vi "Test MFC Step Response.vi"() -> ()   [LabVIEW 2013]
doc: "This VI gets the step response of the 500 SLPM mass flow controller controlling the air flow through the system. It records the pressure readings directly from the static pressure sensor just down stream of the sintered plate in the combustor.\n\nIt can also be used to test the fuel mass flow controllers by selecting the fuel line using the enum on the front panel and then inputting a voltage to the MFC. No pressure sensors are attached to the fuel MFCs."
uses:
  Controls/mfc_enable_boolean_cluster.ctl
  Controls/mfc_voltage_cluster.ctl
  <vilib>/DAQmx/write.llb/DAQmx Write (Digital 1D Bool NChan 1Samp 1Line).vi
  <vilib>/DAQmx/write.llb/DAQmx Write (Analog 1D DBL NChan 1Samp).vi
  <vilib>/DAQmx/read.llb/DAQmx Read (Analog 1D DBL NChan 1Samp).vi
  <vilib>/DAQmx/read.llb/DAQmx Read (Analog 2D DBL NChan NSamp).vi
  <vilib>/DAQmx/miscellaneous.llb/DAQmx Fill In Error Info.vi
  <vilib>/Analysis/NI_AALPro.lvlib
  <resource>/objmgr/daqmx.rc
  <vilib>/ptbypt/NI_PtbyPt.lvlib
panel:
  out "Flame?":bool
  out "Elapsed Time (s)":dbl
  in  "End":bool
  out "Remaining":dbl caption="Time to Shutdown"
  out "Over Temp?":T1 caption="Over Temperature"
  in  "Save Data?":bool
  in  "MFC Voltage":T2 {"Outer" scale=0.0..5.0; "Middle" scale=0.0..5.0; "Pilot" scale=0.0..5.0; "Air" scale=0.0..5.0}
  in  "MFC Enable":T3
  out "Pressure Response":T4(graph)
  in  "Stop Button":bool
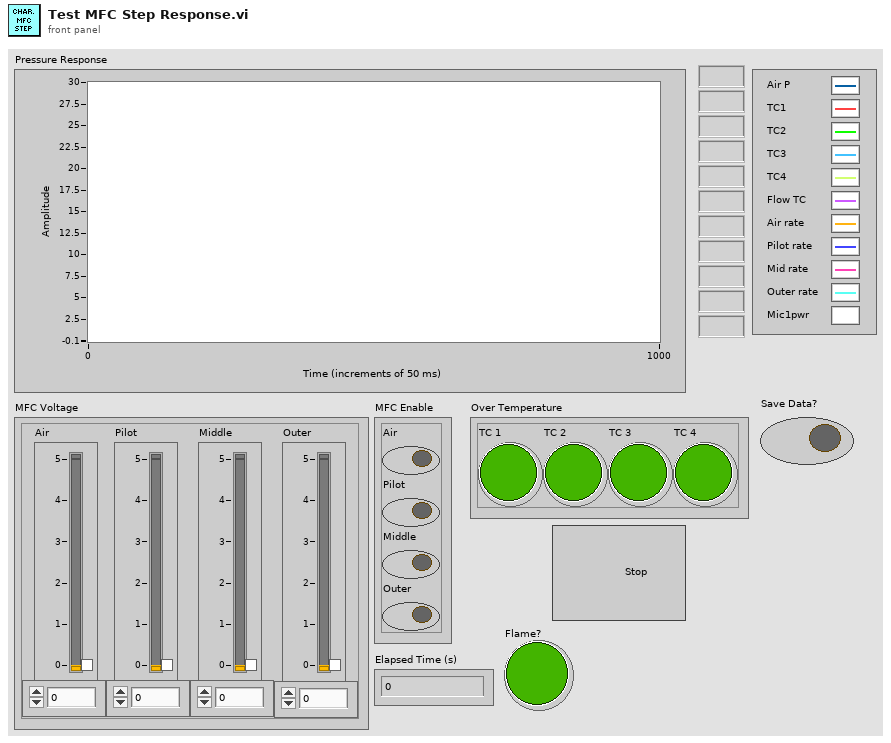
[diagram p1: front panel]
types:
  T1 = cluster{"TC 1":bool, "TC 2":bool, "TC 3":bool, "TC 4":bool}
  T2 = typedef "mfc_voltage_cluster.ctl" = cluster{"Air":dbl, "Pilot":dbl, "Middle":dbl, "Outer":dbl}
  T3 = typedef "mfc_enable_boolean_cluster.ctl" = cluster{"Air":bool, "Pilot":bool, "Middle":bool, "Outer":bool}
  T4 = cluster{"[0]":dbl, "[1]":dbl, "[2]":dbl, "[3]":dbl, "[4]":dbl, "[5]":dbl, "[6]":dbl, "[7]":dbl, "[8]":dbl, "[9]":dbl, "[10]":dbl}
  T5 = enum16{"open", "replace", "create", "open or create", "replace or create", "replace or create with confirmation"}
  T6 = cluster{"[0]":bool, "[1]":bool, "[2]":bool, "[3]":bool}
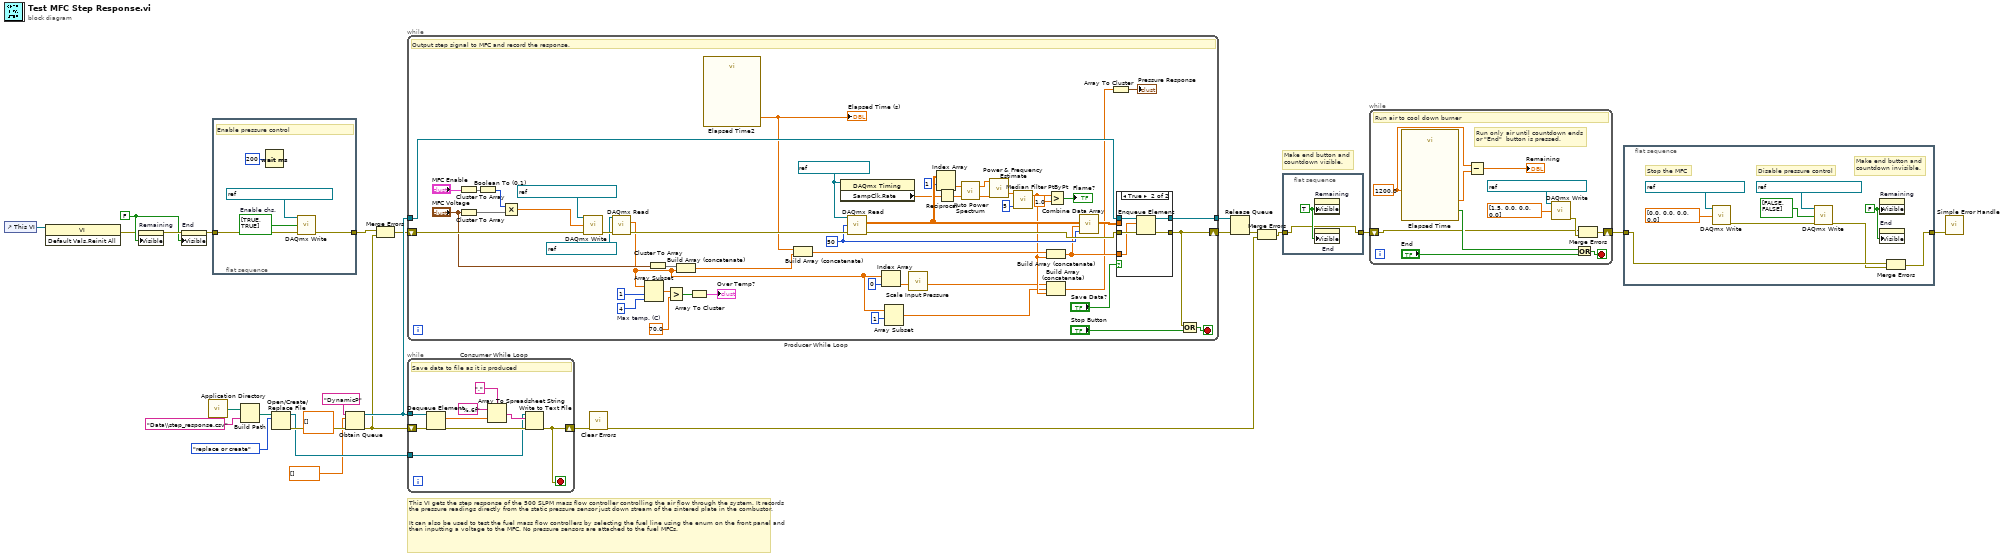
[diagram p0: block diagram]
diagram:
  (unwired) dbl[][] [] ("data")
  w23 = FALSE ("Visible")
  # "Make end button and\ncountdown visible."
  # "This VI gets the step response of the 500 SLPM mass flow controller controlling the air flow through the system. It records the pressure readings directly from the static pressure sensor just down stream of the sintered plate in the combustor.\n\nIt can also be used to test the fuel mass flow controllers by selecting the fuel line using the enum on the front panel and then inputting a voltage to the MFC. No pressure sensors are attached to the fuel MFCs."
  n1 = control-ref of="This VI"() -> (w26:refnum<vi>)
  n2 = invoke class="VI" method="Default Vals.Reinit All"(reference=w26) -> (error out=w18:errorcluster)  [unwired: 2 in, 2 out]
  n3 = property on="Remaining" class="DigNum (strict)"(error in=w18, "Visible"=w23) -> (error out=w25:errorcluster)  [unwired: 1 in, 1 out]
  n4 = property on="End" class="Bool"(error in=w25, "Visible"=w23) -> (error out=w24:errorcluster)  [unwired: 1 in, 1 out]
  n5 = call <vilib>:"Application Directory.vi"() -> ("Application Directory"=w14:path)
  n6 = flat-sequence {
    tunnel: [w29] -> w20
    tunnel: w24 -> [w27]
    frame #0 {
      w28 = bool[] [TRUE, TRUE]  # Enable chs.
      # "Enable pressure control"
      n7 = Wait (ms)(milliseconds to wait=u32 200) -> ()  [unwired: 1 out]
      n8 = call-poly <vilib>:"DAQmx Write.vi"("task/channels in"=refnum<k21> "MFCOutputEnable_S2P0L67", "data"=w28, "error in"=w27) -> ("error out"=w29:errorcluster)  [unwired: 10 in, 2 out]
    }
  }
  n9 = Build Path(base path=w14, name or relative path="Data\\step_response.csv") -> (appended path=w8:path)
  n10 = Open/Create/Replace File(file path (use dialog)=w8, operation (0:open)=T5."replace or create") -> (refnum out=w7:refnum<file>, error out=w9:errorcluster)  [unwired: 4 in, 1 out]
  n11 = Obtain Queue(name (unnamed)="DynamicP", element data type=dbl[] [], error in (no error)=w9) -> (queue out=w21:refnum<queue>, error out=w12:errorcluster)  [unwired: 2 in, 1 out]
  n12 = Merge Errors(w20, w12) -> (w19:errorcluster)
  n13 = while "Producer While Loop" {
    shift-right: [w66] -> w16
    shift-left: w19 -> [w75]
    tunnel: w21 -> [w67]
    tunnel: [w65] -> w15
    stop <- w80 stop-if-true
    w63 = 50 ("number of samples per channel")
    w50 = refnum<k21> "DynP_all_S6AI0-4" ("task/channels in")
    w72 = 70.0  # Max temp. (C)
    # "Output step signal to MFC and record the response."
    n14 = Cluster To Array(cluster="MFC Enable") -> (array=w78:bool[])
    n15 = Cluster To Array(cluster="MFC Voltage") -> (array=w77:dbl[])
    n16 = Boolean To (0,1)(Boolean=w78) -> (0, 1=w76:i16[])
    n17 = Multiply(x=w76, y=w77) -> (x*y=w38:dbl[])
    n18 = call-poly <vilib>:"DAQmx Write.vi"("task/channels in"=refnum<k21> "MFCVoltageOut_S2AO0-3", "data"=w38, "error in"=w75) -> ("error out"=w74:errorcluster)  [unwired: 10 in, 2 out]
    n19 = call-poly <vilib>:"DAQmx Read.vi"("task/channels in"=refnum<k21> "AiTasks_TC_P_S3" ("DAQmx Task Name"), "error in"=w74) -> ("data"=w35:dbl[], "error out"=w71:errorcluster)  [unwired: 11 in, 1 out]
    n20 = Array Subset(array=w35, index=1, length=4) -> (w58:dbl[])
    n21 = Cluster To Array(cluster="MFC Voltage") -> (array=w69:dbl[])
    n22 = Greater?(x=w58, y=w72) -> (0:w57:bool[])
    n23 = Build Array (concatenate)(w69, w35) -> (w60:dbl[])
    n24 = Array To Cluster(array=w57) -> (cluster=→"Over Temp?":T6)
    n25 = call "Elapsed Time2"() -> ("Elapsed Time (s)"=w61:dbl)  [unwired: 12 in, 7 out]
    "Elapsed Time (s)" <- w61
    n26 = Build Array (concatenate)(w61, w60) -> (w55:dbl[])
    n27 = property class="DAQmx Timing"(reference=w50) -> ("SampClk.Rate"=w49:dbl)  [unwired: 1 in, 2 out]
    n28 = call-poly <vilib>:"DAQmx Read.vi"("task/channels in"=w50, "number of samples per channel"=w63, "error in"=w71) -> ("data"=w53:dbl[][], "error out"=w83:errorcluster)  [unwired: 10 in, 1 out]
    n29 = Index Array(array=w35, index=0) -> (element=w36:dbl)
    n30 = Array Subset(array=w35, index=1) -> (w32:dbl[])  [unwired: 1 in]
    n31 = call "Scale Input Pressure.vi"("Pressure (V)"=w36) -> ("Pressure (psi atm)"=w33:dbl)  [unwired: 10 in]
    n32 = Index Array(array=w53, index (row)=1) -> (element=w51:dbl[])  [unwired: 1 in]
    n33 = Reciprocal(x=w49) -> (1/x=w48:dbl)
    n34 = call <vilib>:"Auto Power Spectrum.vi"("dt"=w48, "Signal (V)"=w51) -> ("df"=w46:dbl, "Power Spectrum (V^2 rms)"=w47:dbl[])
    n35 = call <vilib>:"Power & Frequency Estimate.vi"("df"=w46, "Power Spectrum (V^2 rms)"=w47) -> ("est power peak"=w43:dbl)  [unwired: 4 in, 1 out]
    n36 = call <vilib>:"Median Filter PtByPt.vi"("rank"=5, "x"=w43) -> ("Filtered x"=w41:dbl)  [unwired: 2 in, 1 out]
    n37 = Build Array (concatenate)(w55, w41) -> (w45:dbl[])
    n38 = Build Array (concatenate)(w33, w32, w41) -> (w44:dbl[])
    n39 = Greater?(x=w41, y=1.0) -> (0:→"Flame?":bool)
    n40 = call "Combine Data Array.vi"("Num. elements"=w63, "Index data"=w45, "Pressure data"=w53) -> ("All data"=w62:dbl[][])  [unwired: 8 in]
    n41 = Array To Cluster(array=w44) -> (cluster=→"Pressure Response":T4)
    n42 = case shown="True" "Save Data?" {
      tunnel: w83 -> [w85 w90]
      tunnel: w67 -> [w84 w89]
      tunnel: [w85 w88] -> w66
      tunnel: [w84 w87] -> w65
      tunnel: w62 -> [_ _]
      tunnel: w45 -> [_ w86]
      frame False {
      }
      frame True {
        n43 = Enqueue Element(queue=w89, element=w86, error in (no error)=w90) -> (queue out=w87:refnum<queue>, error out=w88:errorcluster)  [unwired: 1 in, 1 out]
      }
    }
    n44 = Or(x=w66, y="Stop Button") -> (x .or. y?=w80:bool)
  }
  n45 = while "Consumer While Loop" {
    tunnel: w21 -> [w98]
    shift-right: [w93] -> w11
    shift-left: w12 -> [w99]
    tunnel: w7 -> [w92]
    stop <- w93 stop-if-true
    # "Save data to file as it is produced"
    n46 = Dequeue Element(queue=w98, error in (no error)=w99) -> (element=w97:dbl[], error out=w94:errorcluster)  [unwired: 1 in, 2 out]
    n47 = Array To Spreadsheet String(delimiter (Tab)=",", array=w97, 3:"%.6f" ("format string")) -> (spreadsheet string=w96:string)
    n48 = Write to Text File(file (use dialog)=w92, text=w96, error in=w94) -> (error out=w93:errorcluster)  [unwired: 1 in, 2 out]
  }
  n49 = call <vilib>:"Clear Errors.vi"("error in (no error)"=w11) -> ("error out"=w10:errorcluster)  [unwired: 6 in]
  n50 = Release Queue(queue=w15, error in (no error)=w16) -> (error out=w17:errorcluster)  [unwired: 1 in, 2 out]
  n51 = Merge Errors(w17, w10) -> (w4:errorcluster)
  n52 = flat-sequence {
    tunnel: w4 -> [w100]
    tunnel: [w100] -> w3
    frame #0 {
      w101 = TRUE ("Visible")
      n53 = property on="Remaining" class="DigNum (strict)"("Visible"=w101) -> ()  [unwired: 2 in, 2 out]
      n54 = property on="End" class="Bool"("Visible"=w101) -> ()  [unwired: 2 in, 2 out]
    }
  }
  n55 = while {
    shift-right: [w104] -> w2
    shift-left: w3 -> [w102]
    stop <- w107 stop-if-true
    w112 = 1200.0 ("Time Target (s)")
    # "Run only air until countdown ends\nor \"End\"  button is pressed."
    # "Run air to cool down burner"
    n56 = call "Elapsed Time"("Time Target (s)"=w112) -> ("Elapsed Time (s)"=w106:dbl, "Time has Elapsed"=w105:bool)  [unwired: 11 in, 6 out]
    n57 = Subtract(x=w112, y=w106) -> (x-y=→"Remaining":dbl)
    n58 = call-poly <vilib>:"DAQmx Write.vi"("task/channels in"=refnum<k21> "MFCVoltageOut_S2AO0-3", "data"=dbl[] [1.5, 0.0, 0.0, 0.0]) -> ("error out"=w103:errorcluster)  [unwired: 11 in, 2 out]
    n59 = Or(x=w105, y="End") -> (x .or. y?=w107:bool)
    n60 = Merge Errors(w102, w103) -> (w104:errorcluster)
  }
  n61 = flat-sequence {
    tunnel: w2 -> [w116]
    tunnel: [w114] -> w1
    frame #0 {
      w121 = FALSE ("Visible")
      # "Make end button and\ncountdown invisible."
      # "Stop the MFC"
      # "Disable pressure control"
      n62 = call-poly <vilib>:"DAQmx Write.vi"("task/channels in"=refnum<k21> "MFCVoltageOut_S2AO0-3", "data"=dbl[] [0.0, 0.0, 0.0, 0.0]) -> ("error out"=w117:errorcluster)  [unwired: 11 in, 2 out]
      n63 = call-poly <vilib>:"DAQmx Write.vi"("task/channels in"=refnum<k21> "MFCOutputEnable_S2P0L67", "data"=bool[] [FALSE, FALSE], "error in"=w117) -> ("error out"=w115:errorcluster)  [unwired: 10 in, 2 out]
      n64 = property on="Remaining" class="DigNum (strict)"("Visible"=w121) -> ()  [unwired: 2 in, 2 out]
      n65 = property on="End" class="Bool"("Visible"=w121) -> ()  [unwired: 2 in, 2 out]
      n66 = Merge Errors(w116, w115) -> (w114:errorcluster)
    }
  }
  n67 = call <vilib>:"Simple Error Handler.vi"("error in (no error)"=w1) -> ()  [unwired: 4 in, 5 out]
